vi "TestExample.vi"() -> ()   [LabVIEW 2020]
uses:
  <vilib>/Instr/_visa.llb/VISA Configure Serial Port (Instr).vi
panel:
  out "error out":errorcluster
  out "Numeric":i32
  in  "stop":bool
  out "read buffer":string
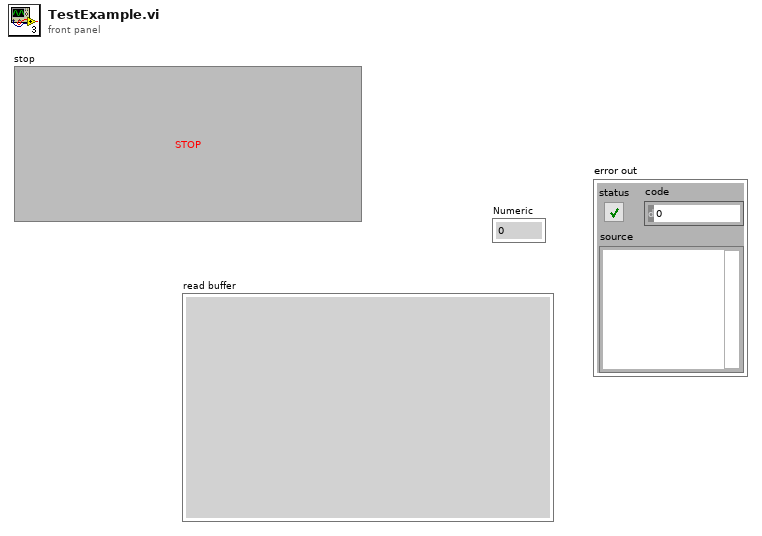
[diagram p1: front panel]
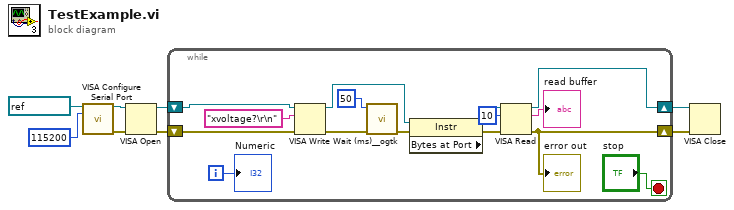
[diagram p0: block diagram]
diagram:
  n1 = call-poly "VISA Configure Serial Port"("VISA resource name"=refnum<visa-resource-name> "COM3", "baud rate (9600)"=u32 115200) -> ("VISA resource name out"=w8:refnum<visa-resource-name>, "error out"=w5:errorcluster)  [unwired: 12 in]
  n2 = VISA Open(error in (no error)=w5, VISA resource name=w8) -> (VISA resource name=w2:refnum<visa-resource-name>, error out=w4:errorcluster)  [unwired: 3 in]
  n3 = while {
    shift-right: [w16] -> w3
    shift-left: w4 -> [w23]
    shift-right: [w21] -> w1
    shift-left: w2 -> [w22]
    i -> [w17]
    stop <- "stop" stop-if-true
    n4 = VISA Write(VISA resource name=w22, write buffer="xvoltage?\r\n", error in (no error)=w23) -> (VISA resource name out=w15:refnum<visa-resource-name>, error out=w12:errorcluster)  [unwired: 1 out]
    n5 = call <userlib>:"Wait (ms)__ogtk.vi"("error in (no error)"=w12, "milliseconds to wait"=u32 50) -> ("error out"=w11:errorcluster)  [unwired: 8 in, 1 out]
    n6 = property class="Instr" props=["Bytes at Port"](reference=w15, error in=w11) -> (reference out=w13:refnum<visa-resource-name>, error out=w14:errorcluster)  [unwired: 1 out]
    n7 = VISA Read(VISA resource name=w13, byte count=u32 10, error in (no error)=w14) -> (VISA resource name out=w21:refnum<visa-resource-name>, read buffer=→"read buffer":string, error out=w16:errorcluster)  [unwired: 1 out]
    "error out" <- w16
    "Numeric" <- w17
  }
  n8 = VISA Close(VISA resource name=w1, error in (no error)=w3) -> ()  [unwired: 1 out]
